vi "ExecuteXML.vi"(8 "error in (no error)":errorcluster, 11 "Auto File Path":path=path "C:/Users/Bendethic/Desktop/AutoRoutineCreator/AutoFiles/1A.txt") -> (0 "error out":errorcluster)   [LabVIEW 2018]
panel:
  out "XML String":string
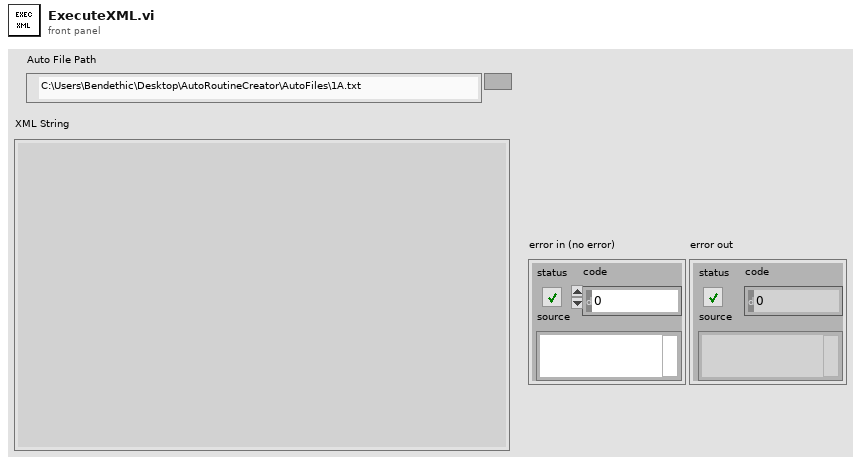
[diagram p1: front panel]
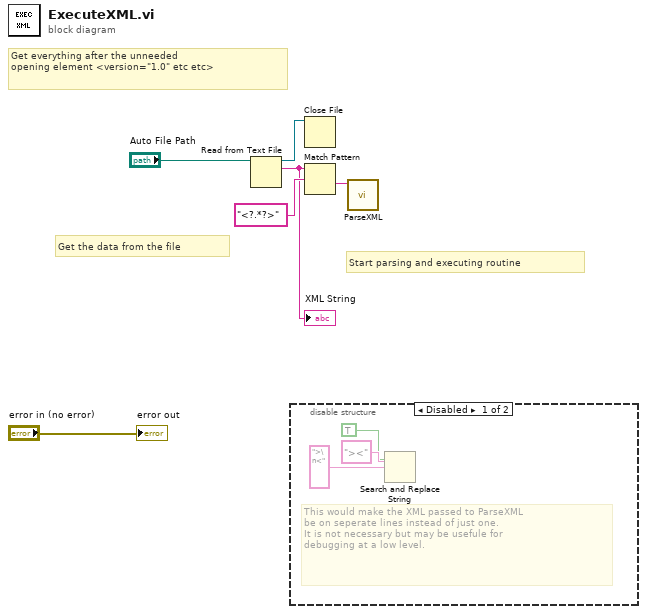
[diagram p0: block diagram]
diagram:
  # "Start parsing and executing routine"
  # "Get everything after the unneeded\nopening element <version=\"1.0\" etc etc>"
  # "Get the data from the file"
  n1 = Read from Text File(file (use dialog)="Auto File Path") -> (refnum out=w2:refnum<file>, text=w3:string)  [unwired: 3 in, 2 out]
  "XML String" <- w3
  n2 = disable-structure shown="Disabled" {
    frame Disabled {
      # "This would make the XML passed to ParseXML\nbe on seperate lines instead of just one.\nIt is not necessary but may be usefule for\ndebugging at a low level."
      n3 = Search and Replace String(replace all?=TRUE ("replace all? (F)"), search string="><", replace string=">\n<" ("replace string (\"\")")) -> ()  [unwired: 5 in, 4 out]
    }
    frame Enabled {
    }
  }
  n4 = Close File(refnum=w2) -> ()  [unwired: 1 in, 2 out]
  n5 = Match Pattern(string=w3, regular expression="<?.*?>") -> (after substring=w1:string)  [unwired: 1 in, 3 out]
  n6 = call "ParseXML.vi"("Node"=w1) -> ()  [unwired: 10 in, 1 out]
  "error out" <- "error in (no error)"
